vi "Obtain Message Queue.vi"(7 "QueueName":string, 8 "ErrorIn":errorcluster) -> (0 "ErrorOut":errorcluster, 3 "Message Queue":refnum<queue>)   [LabVIEW 2016, in "Message Queue.lvlib"]
doc: "Créer une file d'attente avec le type de données du cluster Message."
uses:
  Message Queue.lvlib
  Message Cluster.ctl
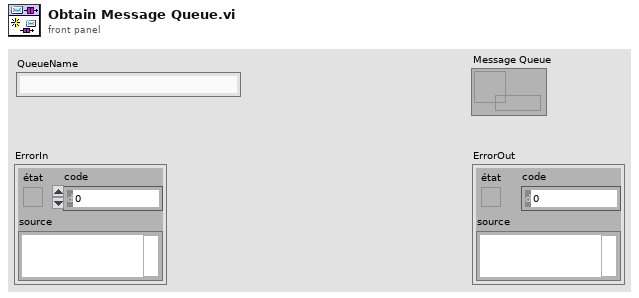
[diagram p1: front panel]
types:
  T1 = typedef "Message Queue.lvlib/Message Cluster.ctl" = cluster{"Message":string, "Données de message":variant}
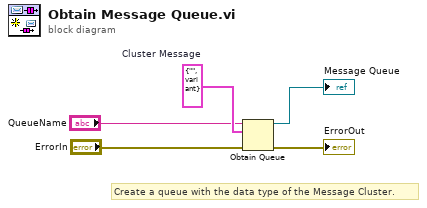
[diagram p0: block diagram]
diagram:
  w5 = T1 {"Message"="", "Données de message"=variant}  # Cluster Message
  # "Create a queue with the data type of the Message Cluster."
  n1 = Obtain Queue(name (unnamed)="QueueName", element data type=w5, error in (no error)="ErrorIn") -> (queue out=→"Message Queue":refnum<queue>, error out=→"ErrorOut":errorcluster)  [unwired: 2 in, 1 out]
